vi "Base Inject Sub.vi"(8 "P2 Disp Speed":dbl=5.0, 9 "P2 Asp Speed":dbl=20.0, 10 "NaOH Steps":u32=500, 11 "FPGA ref in":T1) -> (3 "FPGA ref out":T1)   [LabVIEW 2013]
uses:
  Types Def/FPGA Reference.ctl
  <vilib>/rvi/interface/common/niFpgaWaitOnOcc.vi
  <vilib>/Utility/error.llb/Error Cluster From Error Code.vi
  <vilib>/rvi/errors/niLvFpgaAdjustHostInterfaceError.vi
  <vilib>/rvi/interface/nirviReadWriteControl/nirviReadWriteControl.xnode
  NiFpgaLv.dll
  <vilib>/rvi/interface/Simulation/niFpgaSimulationCallBeginRW.vi
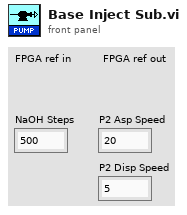
[diagram p1: front panel]
types:
  T1 = typedef "FPGA Reference.ctl" = refnum<k20>
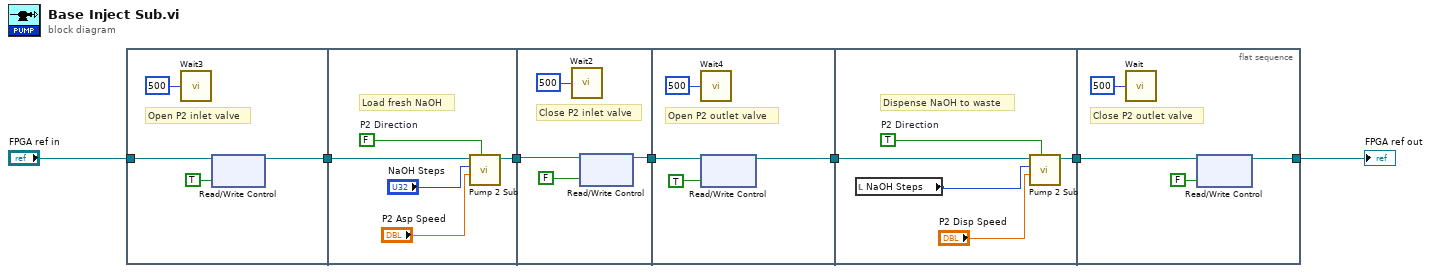
[diagram p0: block diagram]
diagram:
  n1 = flat-sequence {
    tunnel: [w9] -> w7
    tunnel: "FPGA ref in" -> [w8]
    tunnel: w7 -> [w16]
    tunnel: [w13] -> w2
    tunnel: w2 -> [w19]
    tunnel: [w18] -> w1
    tunnel: w1 -> [w22]
    tunnel: [w21] -> w6
    tunnel: w6 -> [w26]
    tunnel: [w28] -> w5
    tunnel: [w32] -> w3
    tunnel: w5 -> [w33]
    frame #0 {
      # "Open P2 inlet valve"
      n2 = call "Wait3"("Count(mSec)"=u32 500) -> ()  [unwired: 1 out]
      n3 = xnode "Read/Write Control"("FPGA VI Reference In"=w8, "VBAsp"=TRUE ("V2-P1 Waste")) -> ("FPGA VI Reference Out"=w9:T1)  [unwired: 1 in, 1 out]
    }
    frame #1 {
      w15 = FALSE  # P2 Direction
      # "Load fresh NaOH"
      n4 = call "Pump 2 Sub.vi"("P2 Direction"=w15, "P2 pps"="P2 Asp Speed", "P2 Steps"="NaOH Steps", "FPGA ref in"=w16) -> ("FPGA ref out"=w13:T1)  [unwired: 6 in, 1 out]
    }
    frame #2 {
      # "Close P2 inlet valve"
      n5 = call "Wait2"("Count(mSec)"=u32 500) -> ()  [unwired: 1 out]
      n6 = xnode "Read/Write Control"("FPGA VI Reference In"=w19, "VBAsp"=FALSE ("V1-Acid")) -> ("FPGA VI Reference Out"=w18:T1)  [unwired: 1 in, 1 out]
    }
    frame #3 {
      # "Open P2 outlet valve"
      n7 = call "Wait4"("Count(mSec)"=u32 500) -> ()  [unwired: 1 out]
      n8 = xnode "Read/Write Control"("FPGA VI Reference In"=w22, "VBDisp"=TRUE ("V2-P1 Waste")) -> ("FPGA VI Reference Out"=w21:T1)  [unwired: 1 in, 1 out]
    }
    frame #4 {
      w29 = TRUE  # P2 Direction
      # "Dispense NaOH to waste"
      n9 = local read "NaOH Steps"() -> (w25:u32)
      n10 = call "Pump 2 Sub.vi"("P2 Direction"=w29, "P2 pps"="P2 Disp Speed", "P2 Steps"=w25, "FPGA ref in"=w26) -> ("FPGA ref out"=w28:T1)  [unwired: 6 in, 1 out]
    }
    frame #5 {
      # "Close P2 outlet valve"
      n11 = call "Wait"("Count(mSec)"=u32 500) -> ()  [unwired: 1 out]
      n12 = xnode "Read/Write Control"("FPGA VI Reference In"=w33, "VBDisp"=FALSE ("V4-P2 Waste")) -> ("FPGA VI Reference Out"=w32:T1)  [unwired: 1 in, 1 out]
    }
  }
  "FPGA ref out" <- w3
